vi "VISJS Viewer.vi"(4 "Extra Scripts":string, 5 "FileDependency In":map{path, T1}(c390), 6 "Options":string, 7 "OpenWebBrowser(False)":bool, 8 "error in":errorcluster, 9 "Embedd VISJS Librarya in HTMl File(False)":bool, 10 "HTMLFilePath":path, 11 "LibraryDependency":map{path, T3}(c390)) -> (0 "error out":errorcluster, 3 "HTMLFileContent":string)   [LabVIEW 2020, in "VISJS Viewer.lvlib"] (continued)
,this.modStack=[],this.blocks=[]}return kd(g,[{key:\"mod\",value:function(){return 0===this.modStack.length?\"normal\":this.modStack[0]}},{key:\"modName\",value:function(){return 0===this.modStack.length?\"normal\":\"mono\"===this.modStack[0]?\"mono\":this.bold&&this.ital?\"boldital\":this.bold?\"bold\":this.ital?\"ital\":void 0}},{key:\"emitBlock\",value:function(){this.spacing&&(this.add(\" \"),this.spacing=!1),this.buffer.length>0&&(this.blocks.push({text:this.buffer,mod:this.modName()}),this.buffer=\"\")}},{key:\"add\",value:function(g){\" \"===g&&(this.spacing=!0),this.spacing&&(this.buffer+=\" \",this.spacing=!1),\" \"!=g&&(this.buffer+=g)}},{key:\"parseWS\",value:function(g){return!!/[ \\t]/.test(g)&&(this.mono?this.add(g):this.spacing=!0,!0)}},{key:\"setTag\",value:function(g){this.emitBlock(),this[g]=!0,this.modStack.unshift(g)}},{key:\"unsetTag\",value:function(g){this.emitBlock(),this[g]=!1,this.modStack.shift()}},{key:\"parseStartTag\",value:function(g,t){return!(this.mono||this[g]||!this.match(t))&&(this.setTag(g),!0)}},{key:\"match\",value:function(g){var t=!(arguments.length>1&&void 0!==arguments[1])||arguments[1],A=lh(this.prepareRegExp(g),2),e=A[0],C=A[1],I=e.test(this.text.substr(this.position,C));return I&&t&&(this.position+=C-1),I}},{key:\"parseEndTag\",value:function(g,t,A){var e=this.mod()===g;return!(!(e=\"mono\"===g?e&&this.mono:e&&!this.mono)||!this.match(t))&&(void 0!==A?(this.position===this.text.length-1||this.match(A,!1))&&this.unsetTag(g):this.unsetTag(g),!0)}},{key:\"replace\",value:function(g,t){return!!this.match(g)&&(this.add(t),this.position+=length-1,!0)}},{key:\"prepareRegExp\",value:function(g){var t,A;if(g instanceof RegExp)A=g,t=1;else{var e=KD[g];A=void 0!==e?e:new RegExp(g),t=g.length}return[A,t]}}]),g}(),XD=function(){function g(t,A,e,C){var I=this;cn(this,g),this.ctx=t,this.parent=A,this.selected=e,this.hover=C;this.lines=new _D((function(g,A){if(void 0===g)return 0;var i=I.parent.getFormattingValues(t,e,C,A),o=0;\"\"!==g&&(o=I.ctx.measureText(g).width);return{width:o,values:i}}))}return kd(g,[{key:\"process\",value:function(g){if(!QD(g))return this.lines.finalize();var t=this.parent.fontOptions;g=(g=g.replace(/\\r\\n/g,\"\\n\")).replace(/\\r/g,\"\\n\");var A=String(g).split(\"\\n\"),e=A.length;if(t.multi)for(var C=0;C<e;C++){var I=this.splitBlocks(A[C],t.multi);if(void 0!==I)if(0!==I.length){if(t.maxWdt>0)for(var i=0;i<I.length;i++){var o=I[i].mod,n=I[i].text;this.splitStringIntoLines(n,o,!0)}else for(var r=0;r<I.length;r++){var s=I[r].mod,a=I[r].text;this.lines.append(a,s)}this.lines.newLine()}else this.lines.newLine(\"\")}else if(t.maxWdt>0)for(var d=0;d<e;d++)this.splitStringIntoLines(A[d]);else for(var h=0;h<e;h++)this.lines.newLine(A[h]);return this.lines.finalize()}},{key:\"decodeMarkupSystem\",value:function(g){var t=\"none\";return\"markdown\"===g||\"md\"===g?t=\"markdown\":!0!==g&&\"html\"!==g||(t=\"html\"),t}},{key:\"splitHtmlBlocks\",value:function(g){for(var t=new HD(g),A=function(g){return!!/&/.test(g)&&(t.replace(t.text,\"&lt;\",\"<\")||t.replace(t.text,\"&amp;\",\"&\")||t.add(\"&\"),!0)};t.position<t.text.length;){var e=t.text.charAt(t.position);t.parseWS(e)||/</.test(e)&&(t.parseStartTag(\"bold\",\"<b>\")||t.parseStartTag(\"ital\",\"<i>\")||t.parseStartTag(\"mono\",\"<code>\")||t.parseEndTag(\"bold\",\"</b>\")||t.parseEndTag(\"ital\",\"</i>\")||t.parseEndTag(\"mono\",\"</code>\"))||A(e)||t.add(e),t.position++}return t.emitBlock(),t.blocks}},{key:\"splitMarkdownBlocks\",value:function(g){for(var t=this,A=new HD(g),e=!0,C=function(g){return!!/\\\\/.test(g)&&(A.position<t.text.length+1&&(A.position++,g=t.text.charAt(A.position),/ \\t/.test(g)?A.spacing=!0:(A.add(g),e=!1)),!0)};A.position<A.text.length;){var I=A.text.charAt(A.position);A.parseWS(I)||C(I)||(e||A.spacing)&&(A.parseStartTag(\"bold\",\"*\")||A.parseStartTag(\"ital\",\"_\")||A.parseStartTag(\"mono\",\"`\"))||A.parseEndTag(\"bold\",\"*\",\"afterBold\")||A.parseEndTag(\"ital\",\"_\",\"afterItal\")||A.parseEndTag(\"mono\",\"`\",\"afterMono\")||(A.add(I),e=!1),A.position++}return A.emitBlock(),A.blocks}},{key:\"splitBlocks\",value:function(g,t){var A=this.decodeMarkupSystem(t);return\"none\"===A?[{text:g,mod:\"normal\"}]:\"markdown\"===A?this.splitMarkdownBlocks(g):\"html\"===A?this.splitHtmlBlocks(g):void 0}},{key:\"overMaxWidth\",value:function(g){var t=this.ctx.measureText(g).width;return this.lines.curWidth()+t>this.parent.fontOptions.maxWdt}},{key:\"getLongestFit\",value:function(g){for(var t=\"\",A=0;A<g.length;){var e=t+(\"\"===t?\"\":\" \")+g[A];if(this.overMaxWidth(e))break;t=e,A++}return A}},{key:\"getLongestFitWord\",value:function(g){for(var t=0;t<g.length&&!this.overMaxWidth(wh(g).call(g,0,t));)t++;return t}},{key:\"splitStringIntoLines\",value:function(g){var t=arguments.length>1&&void 0!==arguments[1]?arguments[1]:\"normal\",A=arguments.length>2&&void 0!==arguments[2]&&arguments[2];this.parent.getFormattingValues(this.ctx,this.selected,this.hover,t);for(var e=(g=(g=g.replace(/^( +)/g,\"$1\\r\")).replace(/([^\\r][^ ]*)( +)/g,\"$1\\r$2\\r\")).split(\"\\r\");e.length>0;){var C=this.getLongestFit(e);if(0===C){var I=e[0],i=this.getLongestFitWord(I);this.lines.newLine(wh(I).call(I,0,i),t),e[0]=wh(I).call(I,i)}else{var o=C;\" \"===e[C-1]?C--:\" \"===e[o]&&o++;var n=wh(e).call(e,0,C).join(\"\");C==e.length&&A?this.lines.append(n,t):this.lines.newLine(n,t),e=wh(e).call(e,o)}}}}]),g}(),JD=[\"bold\",\"ital\",\"boldital\",\"mono\"],qD=function(){function g(t,A){var e=arguments.length>2&&void 0!==arguments[2]&&arguments[2];cn(this,g),this.body=t,this.pointToSelf=!1,this.baseSize=void 0,this.fontOptions={},this.setOptions(A),this.size={top:0,left:0,width:0,height:0,yLine:0},this.isEdgeLabel=e}return kd(g,[{key:\"setOptions\",value:function(g){if(this.elementOptions=g,this.initFontOptions(g.font),QD(g.label)?this.labelDirty=!0:g.label=void 0,void 0!==g.font&&null!==g.font)if(\"string\"==typeof g.font)this.baseSize=this.fontOptions.size;else if(\"object\"===yd(g.font)){var t=g.font.size;void 0!==t&&(this.baseSize=t)}}},{key:\"initFontOptions\",value:function(t){var A=this;tv(JD,(function(g){A.fontOptions[g]={}})),g.parseFontString(this.fontOptions,t)?this.fontOptions.vadjust=0:tv(t,(function(g,t){null!=g&&\"object\"!==yd(g)&&(A.fontOptions[t]=g)}))}},{key:\"constrain\",value:function(g){var t={constrainWidth:!1,maxWdt:-1,minWdt:-1,constrainHeight:!1,minHgt:-1,valign:\"middle\"},A=lv(g,\"widthConstraint\");if(\"number\"==typeof A)t.maxWdt=Number(A),t.minWdt=Number(A);else if(\"object\"===yd(A)){var e=lv(g,[\"widthConstraint\",\"maximum\"]);\"number\"==typeof e&&(t.maxWdt=Number(e));var C=lv(g,[\"widthConstraint\",\"minimum\"]);\"number\"==typeof C&&(t.minWdt=Number(C))}var I=lv(g,\"heightConstraint\");if(\"number\"==typeof I)t.minHgt=Number(I);else if(\"object\"===yd(I)){var i=lv(g,[\"heightConstraint\",\"minimum\"]);\"number\"==typeof i&&(t.minHgt=Number(i));var o=lv(g,[\"heightConstraint\",\"valign\"]);\"string\"==typeof o&&(\"top\"!==o&&\"bottom\"!==o||(t.valign=o))}return t}},{key:\"update\",value:function(g,t){this.setOptions(g,!0),this.propagateFonts(t),qf(this.fontOptions,this.constrain(t)),this.fontOptions.chooser=YD(\"label\",t)}},{key:\"adjustSizes\",value:function(g){var t=g?g.right+g.left:0;this.fontOptions.constrainWidth&&(this.fontOptions.maxWdt-=t,this.fontOptions.minWdt-=t);var A=g?g.top+g.bottom:0;this.fontOptions.constrainHeight&&(this.fontOptions.minHgt-=A)}},{key:\"addFontOptionsToPile\",value:function(g,t){for(var A=0;A<t.length;++A)this.addFontToPile(g,t[A])}},{key:\"addFontToPile\",value:function(g,t){if(void 0!==t&&void 0!==t.font&&null!==t.font){var A=t.font;g.push(A)}}},{key:\"getBasicOptions\",value:function(t){for(var A={},e=0;e<t.length;++e){var C=t[e],I={};g.parseFontString(I,C)&&(C=I),tv(C,(function(g,t){void 0!==g&&(Object.prototype.hasOwnProperty.call(A,t)||(-1!==Xc(JD).call(JD,t)?A[t]={}:A[t]=g))}))}return A}},{key:\"getFontOption\",value:function(t,A,e){for(var C,I=0;I<t.length;++I){var i=t[I];if(Object.prototype.hasOwnProperty.call(i,A)){if(null==(C=i[A]))continue;var o={};if(g.parseFontString(o,C)&&(C=o),Object.prototype.hasOwnProperty.call(C,e))return C[e]}}if(Object.prototype.hasOwnProperty.call(this.fontOptions,e))return this.fontOptions[e];throw new Error(\"Did not find value for multi-font for property: '\"+e+\"'\")}},{key:\"getFontOptions\",value:function(g,t){for(var A={},e=[\"color\",\"size\",\"face\",\"mod\",\"vadjust\"],C=0;C<e.length;++C){var I=e[C];A[I]=this.getFontOption(g,t,I)}return A}},{key:\"propagateFonts\",value:function(g){var t=this,A=[];this.addFontOptionsToPile(A,g),this.fontOptions=this.getBasicOptions(A);for(var e=function(){var g=JD[C],e=t.fontOptions[g];tv(t.getFontOptions(A,g),(function(g,t){e[t]=g})),e.size=Number(e.size),e.vadjust=Number(e.vadjust)},C=0;C<JD.length;++C)e()}},{key:\"draw\",value:function(g,t,A,e,C){var I=arguments.length>5&&void 0!==arguments[5]?arguments[5]:\"middle\";if(void 0!==this.elementOptions.label){var i=this.fontOptions.size*this.body.view.scale;this.elementOptions.label&&i<this.elementOptions.scaling.label.drawThreshold-1||(i>=this.elementOptions.scaling.label.maxVisible&&(i=Number(this.elementOptions.scaling.label.maxVisible)/this.body.view.scale),this.calculateLabelSize(g,e,C,t,A,I),this._drawBackground(g),this._drawText(g,t,this.size.yLine,I,i))}}},{key:\"_drawBackground\",value:function(g){if(void 0!==this.fontOptions.background&&\"none\"!==this.fontOptions.background){g.fillStyle=this.fontOptions.background;var t=this.getSize();g.fillRect(t.left,t.top,t.width,t.height)}}},{key:\"_drawText\",value:function(g,t,A){var e=arguments.length>3&&void 0!==arguments[3]?arguments[3]:\"middle\",C=arguments.length>4?arguments[4]:void 0,I=lh(this._setAlignment(g,t,A,e),2);t=I[0],A=I[1],g.textAlign=\"left\",t-=this.size.width/2,this.fontOptions.valign&&this.size.height>this.size.labelHeight&&(\"top\"===this.fontOptions.valign&&(A-=(this.size.height-this.size.labelHeight)/2),\"bottom\"===this.fontOptions.valign&&(A+=(this.size.height-this.size.labelHeight)/2));for(var i=0;i<this.lineCount;i++){var o=this.lines[i];if(o&&o.blocks){var n=0;this.isEdgeLabel||\"center\"===this.fontOptions.align?n+=(this.size.width-o.width)/2:\"right\"===this.fontOptions.align&&(n+=this.size.width-o.width);for(var r=0;r<o.blocks.length;r++){var s=o.blocks[r];g.font=s.font;var a=lh(this._getColor(s.color,C,s.strokeColor),2),d=a[0],h=a[1];s.strokeWidth>0&&(g.lineWidth=s.strokeWidth,g.strokeStyle=h,g.lineJoin=\"round\"),g.fillStyle=d,s.strokeWidth>0&&g.strokeText(s.text,t+n,A+s.vadjust),g.fillText(s.text,t+n,A+s.vadjust),n+=s.width}A+=o.height}}}},{key:\"_setAlignment\",value:function(g,t,A,e){if(this.isEdgeLabel&&\"horizontal\"!==this.fontOptions.align&&!1===this.pointToSelf){t=0,A=0;\"top\"===this.fontOptions.align?(g.textBaseline=\"alphabetic\",A-=4):\"bottom\"===this.fontOptions.align?(g.textBaseline=\"hanging\",A+=4):g.textBaseline=\"middle\"}else g.textBaseline=e;return[t,A]}},{key:\"_getColor\",value:function(g,t,A){var e=g||\"#000000\",C=A||\"#ffffff\";if(t<=this.elementOptions.scaling.label.drawThreshold){var I=Math.max(0,Math.min(1,1-(this.elementOptions.scaling.label.drawThreshold-t)));e=ev(e,I),C=ev(C,I)}return[e,C]}},{key:\"getTextSize\",value:function(g){var t=arguments.length>1&&void 0!==arguments[1]&&arguments[1],A=arguments.length>2&&void 0!==arguments[2]&&arguments[2];return this._processLabel(g,t,A),{width:this.size.width,height:this.size.height,lineCount:this.lineCount}}},{key:\"getSize\",value:function(){var g=this.size.left,t=this.size.top-1;if(this.isEdgeLabel){var A=.5*-this.size.width;switch(this.fontOptions.align){case\"middle\":g=A,t=.5*-this.size.height;break;case\"top\":g=A,t=-(this.size.height+2);break;case\"bottom\":g=A,t=2}}return{left:g,top:t,width:this.size.width,height:this.size.height}}},{key:\"calculateLabelSize\",value:function(g,t,A){var e=arguments.length>3&&void 0!==arguments[3]?arguments[3]:0,C=arguments.length>4&&void 0!==arguments[4]?arguments[4]:0,I=arguments.length>5&&void 0!==arguments[5]?arguments[5]:\"middle\";this._processLabel(g,t,A),this.size.left=e-.5*this.size.width,this.size.top=C-.5*this.size.height,this.size.yLine=C+.5*(1-this.lineCount)*this.fontOptions.size,\"hanging\"===I&&(this.size.top+=.5*this.fontOptions.size,this.size.top+=4,this.size.yLine+=4)}},{key:\"getFormattingValues\",value:function(g,t,A,e){var C=function(g,t,A){return\"normal\"===t?\"mod\"===A?\"\":g[A]:void 0!==g[t][A]?g[t][A]:g[A]},I={color:C(this.fontOptions,e,\"color\"),size:C(this.fontOptions,e,\"size\"),face:C(this.fontOptions,e,\"face\"),mod:C(this.fontOptions,e,\"mod\"),vadjust:C(this.fontOptions,e,\"vadjust\"),strokeWidth:this.fontOptions.strokeWidth,strokeColor:this.fontOptions.strokeColor};(t||A)&&(\"normal\"===e&&!0===this.fontOptions.chooser&&this.elementOptions.labelHighlightBold?I.mod=\"bold\":\"function\"==typeof this.fontOptions.chooser&&this.fontOptions.chooser(I,this.elementOptions.id,t,A));var i=\"\";return void 0!==I.mod&&\"\"!==I.mod&&(i+=I.mod+\" \"),i+=I.size+\"px \"+I.face,g.font=i.replace(/\"/g,\"\"),I.font=g.font,I.height=I.size,I}},{key:\"differentState\",value:function(g,t){return g!==this.selectedState||t!==this.hoverState}},{key:\"_processLabelText\",value:function(g,t,A,e){return new XD(g,this,t,A).process(e)}},{key:\"_processLabel\",value:function(g,t,A){if(!1!==this.labelDirty||this.differentState(t,A)){var e=this._processLabelText(g,t,A,this.elementOptions.label);this.fontOptions.minWdt>0&&e.width<this.fontOptions.minWdt&&(e.width=this.fontOptions.minWdt),this.size.labelHeight=e.height,this.fontOptions.minHgt>0&&e.height<this.fontOptions.minHgt&&(e.height=this.fontOptions.minHgt),this.lines=e.lines,this.lineCount=e.lines.length,this.size.width=e.width,this.size.height=e.height,this.selectedState=t,this.hoverState=A,this.labelDirty=!1}}},{key:\"visible\",value:function(){return 0!==this.size.width&&0!==this.size.height&&void 0!==this.elementOptions.label&&!(this.fontOptions.size*this.body.view.scale<this.elementOptions.scaling.label.drawThreshold-1)}}],[{key:\"parseFontString\",value:function(g,t){if(!t||\"string\"!=typeof t)return!1;var A=t.split(\" \");return g.size=+A[0].replace(\"px\",\"\"),g.face=A[1],g.color=A[2],!0}}]),g}(),$D=function(){function g(t,A,e){cn(this,g),this.body=A,this.labelModule=e,this.setOptions(t),this.top=void 0,this.left=void 0,this.height=void 0,this.width=void 0,this.radius=void 0,this.margin=void 0,this.refreshNeeded=!0,this.boundingBox={top:0,left:0,right:0,bottom:0}}return kd(g,[{key:\"setOptions\",value:function(g){this.options=g}},{key:\"_setMargins\",value:function(g){this.margin={},this.options.margin&&(\"object\"==yd(this.options.margin)?(this.margin.top=this.options.margin.top,this.margin.right=this.options.margin.right,this.margin.bottom=this.options.margin.bottom,this.margin.left=this.options.margin.left):(this.margin.top=this.options.margin,this.margin.right=this.options.margin,this.margin.bottom=this.options.margin,this.margin.left=this.options.margin)),g.adjustSizes(this.margin)}},{key:\"_distanceToBorder\",value:function(g,t){var A=this.options.borderWidth;return g&&this.resize(g),Math.min(Math.abs(this.width/2/Math.cos(t)),Math.abs(this.height/2/Math.sin(t)))+A}},{key:\"enableShadow\",value:function(g,t){t.shadow&&(g.shadowColor=t.shadowColor,g.shadowBlur=t.shadowSize,g.shadowOffsetX=t.shadowX,g.shadowOffsetY=t.shadowY)}},{key:\"disableShadow\",value:function(g,t){t.shadow&&(g.shadowColor=\"rgba(0,0,0,0)\",g.shadowBlur=0,g.shadowOffsetX=0,g.shadowOffsetY=0)}},{key:\"enableBorderDashes\",value:function(g,t){if(!1!==t.borderDashes)if(void 0!==g.setLineDash){var A=t.borderDashes;!0===A&&(A=[5,15]),g.setLineDash(A)}else console.warn(\"setLineDash is not supported in this browser. The dashed borders cannot be used.\"),this.options.shapeProperties.borderDashes=!1,t.borderDashes=!1}},{key:\"disableBorderDashes\",value:function(g,t){!1!==t.borderDashes&&(void 0!==g.setLineDash?g.setLineDash([0]):(console.warn(\"setLineDash is not supported in this browser. The dashed borders cannot be used.\"),this.options.shapeProperties.borderDashes=!1,t.borderDashes=!1))}},{key:\"needsRefresh\",value:function(g,t){return!0===this.refreshNeeded?(this.refreshNeeded=!1,!0):void 0===this.width||this.labelModule.differentState(g,t)}},{key:\"initContextForDraw\",value:function(g,t){var A=t.borderWidth/this.body.view.scale;g.lineWidth=Math.min(this.width,A),g.strokeStyle=t.borderColor,g.fillStyle=t.color}},{key:\"performStroke\",value:function(g,t){var A=t.borderWidth/this.body.view.scale;g.save(),A>0&&(this.enableBorderDashes(g,t),g.stroke(),this.disableBorderDashes(g,t)),g.restore()}},{key:\"performFill\",value:function(g,t){g.save(),g.fillStyle=t.color,this.enableShadow(g,t),Bu(g).call(g),this.disableShadow(g,t),g.restore(),this.performStroke(g,t)}},{key:\"_addBoundingBoxMargin\",value:function(g){this.boundingBox.left-=g,this.boundingBox.top-=g,this.boundingBox.bottom+=g,this.boundingBox.right+=g}},{key:\"_updateBoundingBox\",value:function(g,t,A,e,C){void 0!==A&&this.resize(A,e,C),this.left=g-this.width/2,this.top=t-this.height/2,this.boundingBox.left=this.left,this.boundingBox.top=this.top,this.boundingBox.bottom=this.top+this.height,this.boundingBox.right=this.left+this.width}},{key:\"updateBoundingBox\",value:function(g,t,A,e,C){this._updateBoundingBox(g,t,A,e,C)}},{key:\"getDimensionsFromLabel\",value:function(g,t,A){this.textSize=this.labelModule.getTextSize(g,t,A);var e=this.textSize.width,C=this.textSize.height;return 0===e&&(e=14,C=14),{width:e,height:C}}}]),g}();function gN(g){var t=function(){if(\"undefined\"==typeof Reflect||!MT)return!1;if(MT.sham)return!1;if(\"function\"==typeof Proxy)return!0;try{return Boolean.prototype.valueOf.call(MT(Boolean,[],(function(){}))),!0}catch(g){return!1}}();return function(){var A,e=nb(g);if(t){var C=nb(this).constructor;A=MT(e,arguments,C)}else A=e.apply(this,arguments);return Ib(this,A)}}var tN=function(g){Cb(A,g);var t=gN(A);function A(g,e,C){var I;return cn(this,A),(I=t.call(this,g,e,C))._setMargins(C),I}return kd(A,[{key:\"resize\",value:function(g){var t=arguments.length>1&&void 0!==arguments[1]?arguments[1]:this.selected,A=arguments.length>2&&void 0!==arguments[2]?arguments[2]:this.hover;if(this.needsRefresh(t,A)){var e=this.getDimensionsFromLabel(g,t,A);this.width=e.width+this.margin.right+this.margin.left,this.height=e.height+this.margin.top+this.margin.bottom,this.radius=this.width/2}}},{key:\"draw\",value:function(g,t,A,e,C,I){this.resize(g,e,C),this.left=t-this.width/2,this.top=A-this.height/2,this.initContextForDraw(g,I),Ve(g,this.left,this.top,this.width,this.height,I.borderRadius),this.performFill(g,I),this.updateBoundingBox(t,A,g,e,C),this.labelModule.draw(g,this.left+this.textSize.width/2+this.margin.left,this.top+this.textSize.height/2+this.margin.top,e,C)}},{key:\"updateBoundingBox\",value:function(g,t,A,e,C){this._updateBoundingBox(g,t,A,e,C);var I=this.options.shapeProperties.borderRadius;this._addBoundingBoxMargin(I)}},{key:\"distanceToBorder\",value:function(g,t){g&&this.resize(g);var A=this.options.borderWidth;return Math.min(Math.abs(this.width/2/Math.cos(t)),Math.abs(this.height/2/Math.sin(t)))+A}}]),A}($D);function AN(g){var t=function(){if(\"undefined\"==typeof Reflect||!MT)return!1;if(MT.sham)return!1;if(\"function\"==typeof Proxy)return!0;try{return Boolean.prototype.valueOf.call(MT(Boolean,[],(function(){}))),!0}catch(g){return!1}}();return function(){var A,e=nb(g);if(t){var C=nb(this).constructor;A=MT(e,arguments,C)}else A=e.apply(this,arguments);return Ib(this,A)}}var eN=function(g){Cb(A,g);var t=AN(A);function A(g,e,C){var I;return cn(this,A),(I=t.call(this,g,e,C)).labelOffset=0,I.selected=!1,I}return kd(A,[{key:\"setOptions\",value:function(g,t,A){this.options=g,void 0===t&&void 0===A||this.setImages(t,A)}},{key:\"setImages\",value:function(g,t){t&&this.selected?(this.imageObj=t,this.imageObjAlt=g):(this.imageObj=g,this.imageObjAlt=t)}},{key:\"switchImages\",value:function(g){var t=g&&!this.selected||!g&&this.selected;
